vi "메인.vi"() -> ()   [LabVIEW 2021]
uses:
  <vilib>/Utility/miscctls.llb/LVPointTypeDef.ctl
  ctl/AI.ctl
  ctl/RS232.ctl
  ctl/DB.ctl
  ctl/SM.ctl
  ctl/CNN.ctl
  <vilib>/userDefined/High Color/IMAQdx.ctl
  <vilib>/Utility/sysdir.llb/System Directory Type.ctl
  <vilib>/DAQmx/read.llb/DAQmx Read (Analog 1D Wfm NChan NSamp).vi
  <vilib>/Analysis/baseanly.llb/Mean (DBL).vi
  <vilib>/Utility/file.llb/Write Delimited Spreadsheet (DBL).vi
  <vilib>/addons/database/Connection.llb/DB Tools Open Connec (String).vi
  <vilib>/Instr/_visa.llb/VISA Configure Serial Port (Instr).vi
  <vilib>/DAQmx/create/channels.llb/DAQmx Create Channel (AI-Voltage-Basic).vi
  <vilib>/DAQmx/configure/timing.llb/DAQmx Timing (Sample Clock).vi
  <vilib>/DAQmx/miscellaneous.llb/DAQmx Fill In Error Info.vi
  <vilib>/Analysis/NI_AALBase.lvlib
  <vilib>/vision/driver/NI_Vision_Acquisition_Software.lvlib
  <vilib>/addons/database/NI_Database_API.lvlib
panel:
  out "원소":i16 format="%.0f ℃"
  out "온도":i16(slide) scale=0.0..100.0
  out "Image 2":T1(plugin-control)
  in  "정지":bool
  in  "측정 시작":bool
  out "CNN Result":string[](array[string])
  out "Factory 상태":string
  in  "여러 열 리스트박스":i32(listbox)
  out "Image":T1(plugin-control)
  out "거리센서":waveform(dbl)(graph)
  out "기울기 그래프":waveform(dbl)[](graph)
  out "가속도 그래프":waveform(dbl)(graph)
  # "Smart Factory Management System"
  # "Factory State"
  # "Accelometer"
  # "Gradient"
  # "Distance"
  # "Object State"
  # "Temperature"
  # "Real Time Image"
  # "Captured Image"
  # "Result Table"
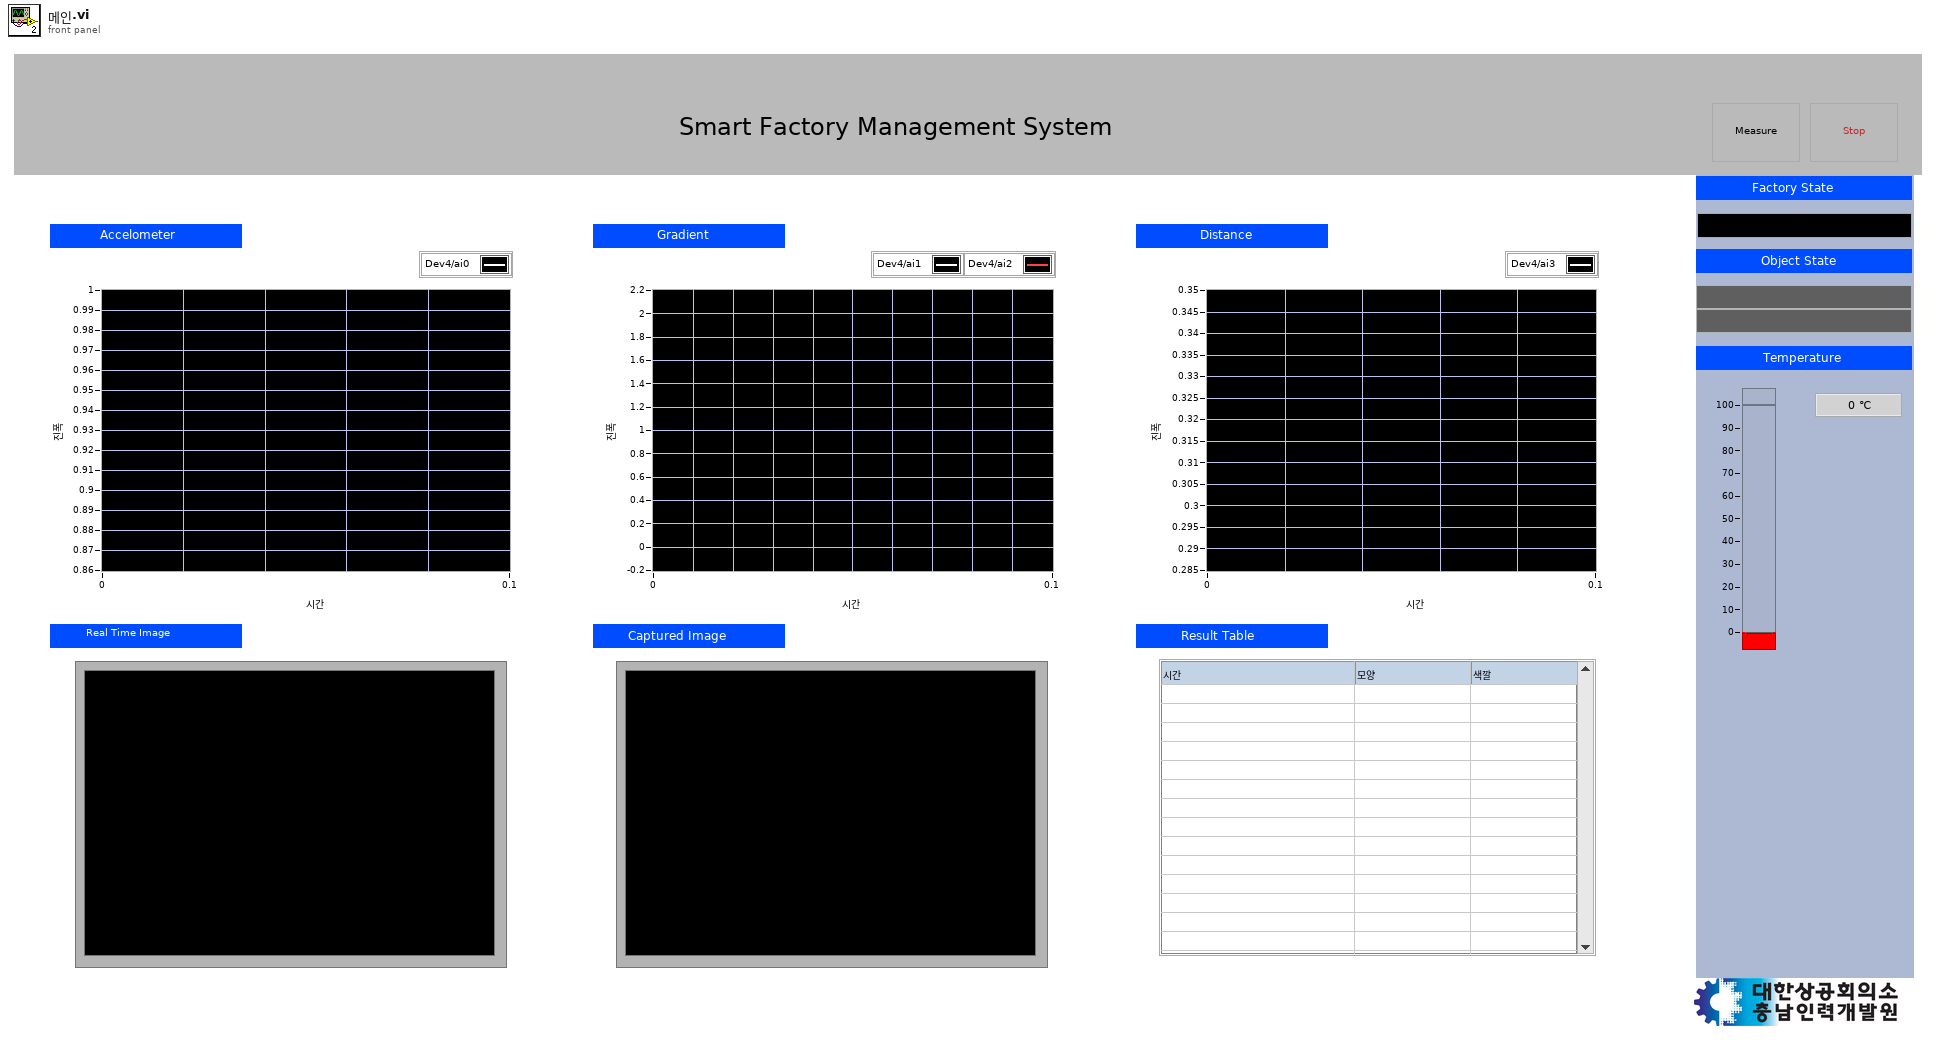
[diagram p1: front panel]
types:
  T1 = typedef "IMAQ Image.ctl" = refnum<image>
  T2 = typedef "LVPointTypeDef.ctl" = cluster{"Horizontal":i16, "Vertical":i16}
  T3 = cluster{"메인":refnum<queue>, "AI":refnum<queue>, "RS-232":refnum<queue>, "비전":refnum<queue>, "DB":refnum<queue>, "SM":refnum<queue>, "CNN":refnum<queue>}
  T4 = typedef "CNN.ctl" = cluster{"상태":enum16{"CNN 통신", "프로그램정지"}, "값":variant}
  T5 = typedef "SM.ctl" = cluster{"상태":enum16{"SM 통신", "프로그램정지"}, "값":variant}
  T6 = typedef "DB.ctl" = cluster{"상태":enum16{"초기화", "설정", "값 쓰기", "에러쓰기", "닫기", "프로그램정지"}, "값":variant}
  T7 = typedef "비전.ctl" = cluster{"상태":enum16{"초기화", "설정", "상시읽기", "트리거읽기", "닫기", "프로그램정지"}, "값":variant}
  T8 = typedef "RS232.ctl" = cluster{"상태":enum16{"초기화", "설정", "읽기", "닫기", "프로그램정지"}, "값":variant}
  T9 = typedef "AI.ctl" = cluster{"상태":enum16{"초기화", "설정", "읽기", "닫기", "프로그램정지"}, "값":variant}
  T10 = typedef "메인.ctl" = cluster{"상태":enum16{"초기화", "프로그램정지"}, "값":variant}
  T11 = enum16{"초기화", "설정", "값 쓰기", "에러쓰기", "닫기", "프로그램정지"}
  T12 = typedef "NI_Database_API.lvlib/Conn ObjectReference.ctl" = refnum<k1>
  T13 = cluster{"[0]":string, "[1]":string, "[2]":string}
  T14 = enum16{"Standard", "Buffered", "CRLF", "Immediate"}
  T15 = typedef "IMAQdx.ctl" = refnum<k21>
  T16 = enum16{"초기화", "설정", "상시읽기", "트리거읽기", "닫기", "프로그램정지"}
  T17 = typedef "System Directory Type.ctl" = i32
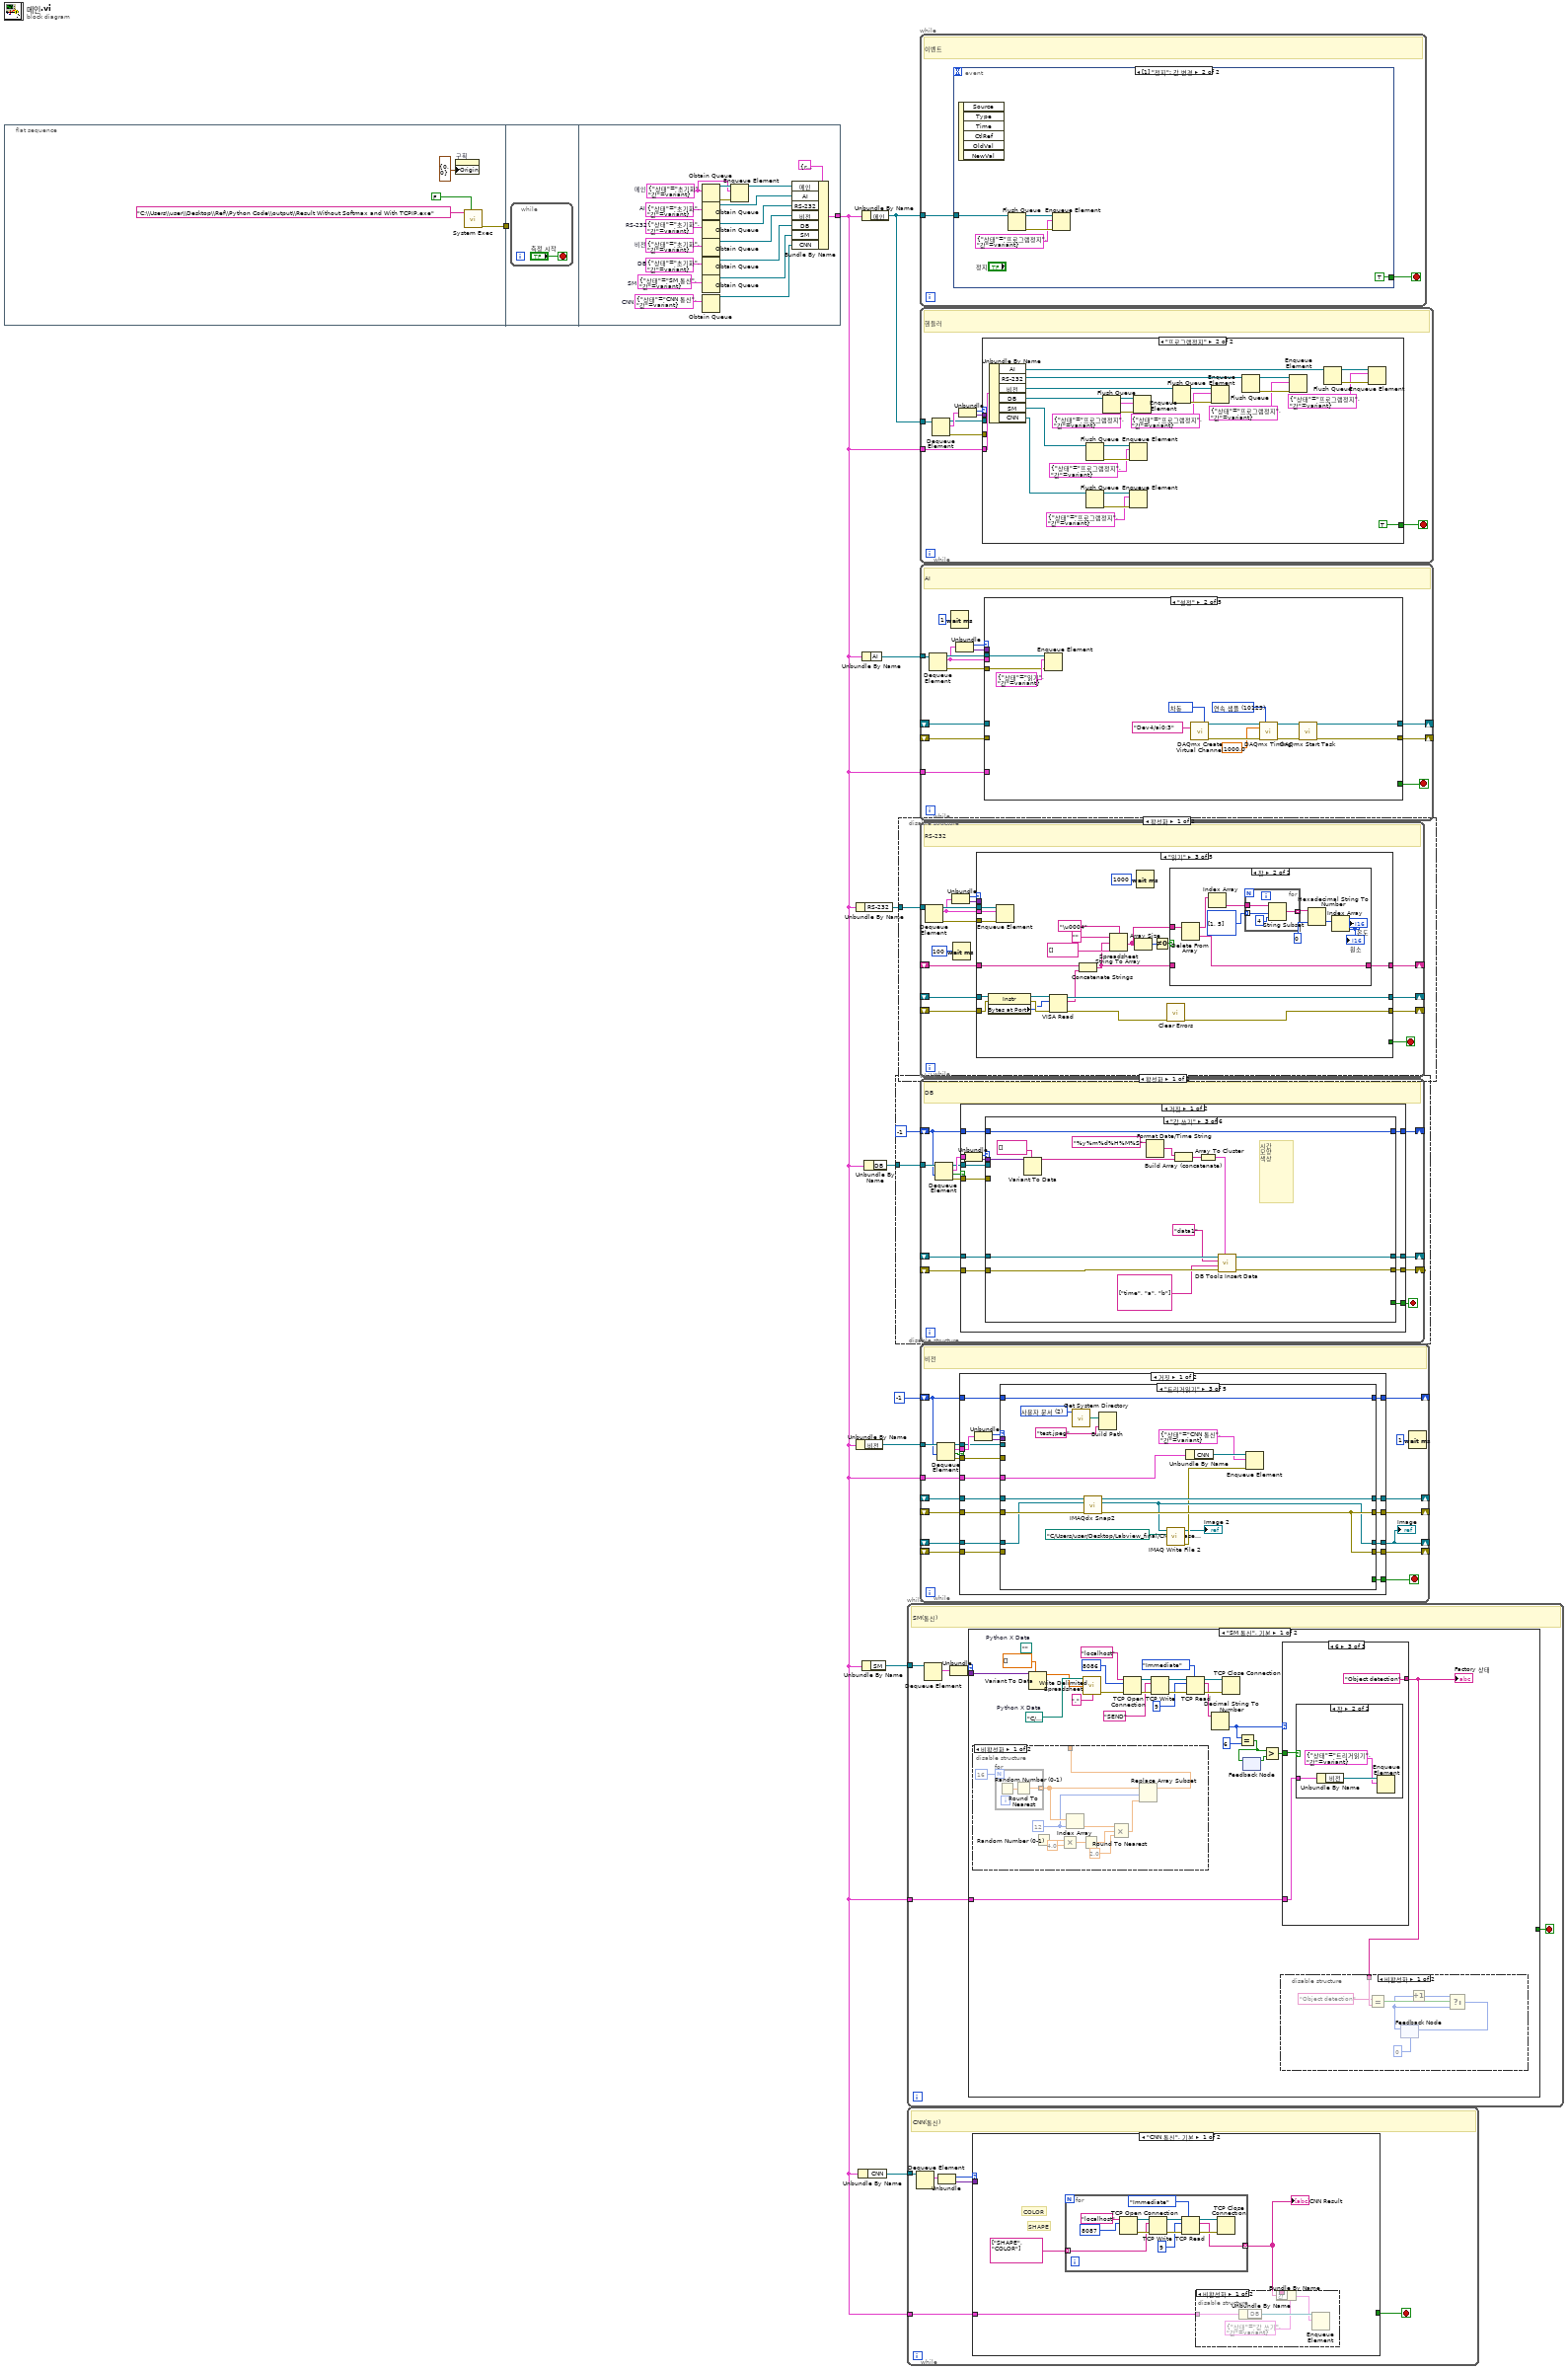
[diagram p0: block diagram]
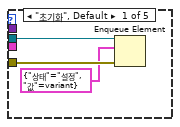
[diagram p2: hidden frame]
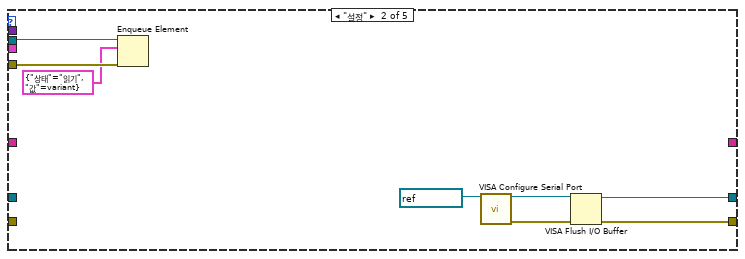
[diagram p3: hidden frame]
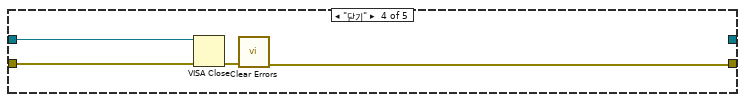
[diagram p5: hidden frame]
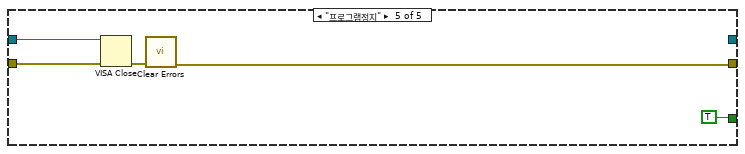
[diagram p6: hidden frame]
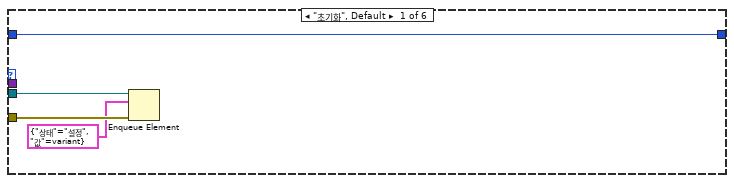
[diagram p8: hidden frame]
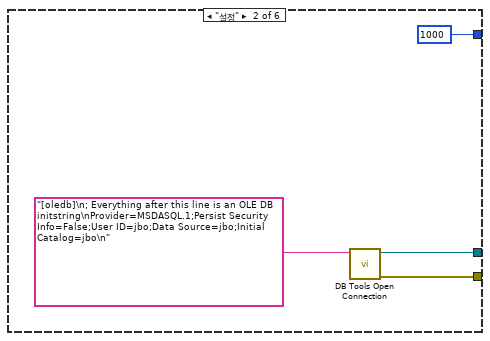
[diagram p9: hidden frame]
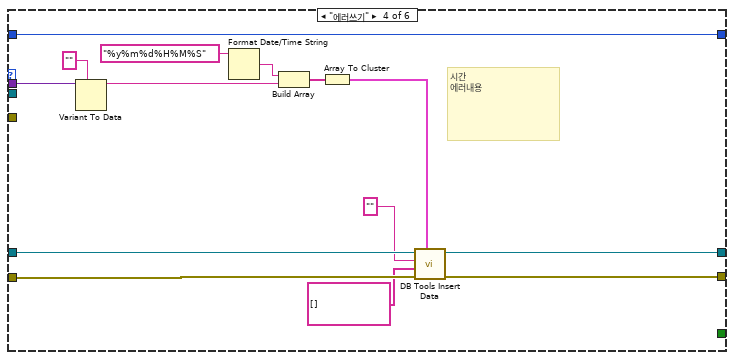
[diagram p10: hidden frame]
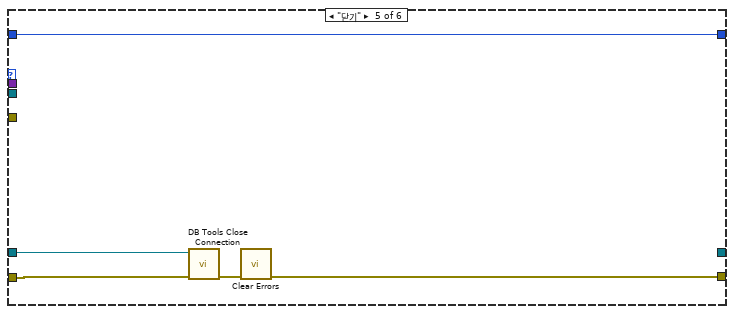
[diagram p11: hidden frame]
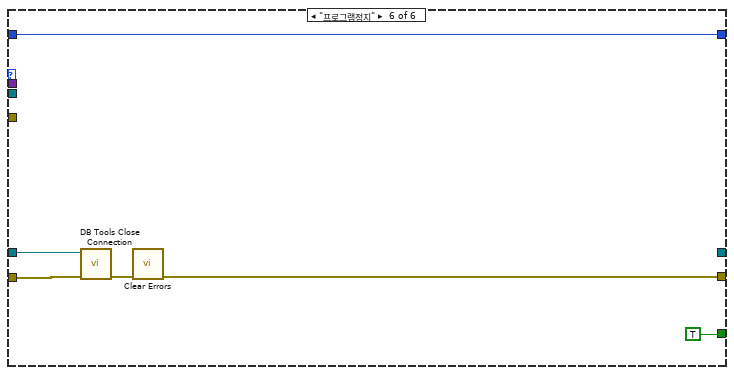
[diagram p12: hidden frame]
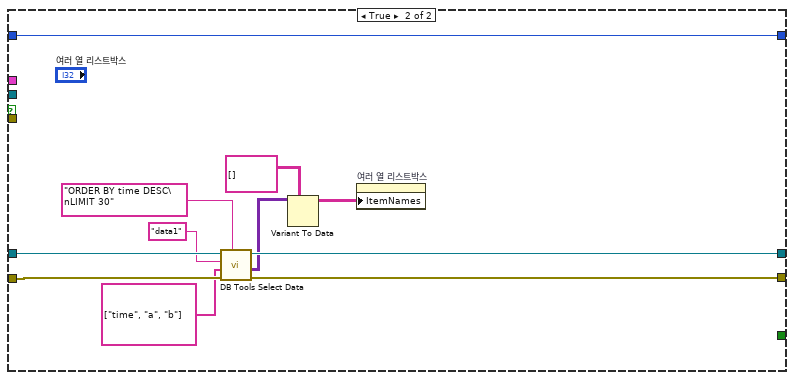
[diagram p13: hidden frame]
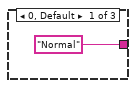
[diagram p17: hidden frame]
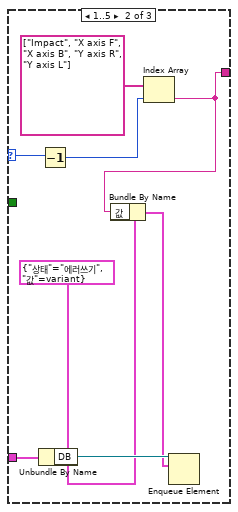
[diagram p18: hidden frame]
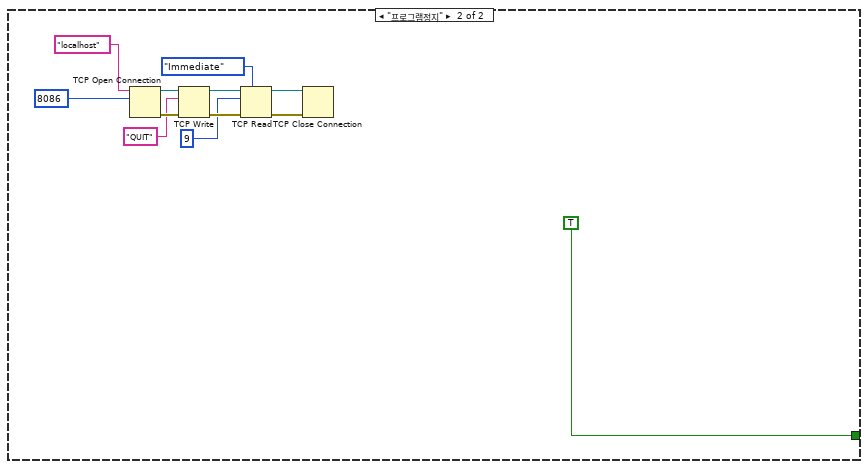
[diagram p20: hidden frame]
diagram:
  n1 = flat-sequence {
    tunnel: [w14] -> w1
    tunnel: w1 -> [_]
    tunnel: [w16] -> w2
    frame #0 {
      n2 = property on="구획" class="Pane"("Origin"=T2 {"Horizontal"=0, "Vertical"=0} ("원점")) -> ()  [unwired: 2 in, 2 out]
      n3 = call <vilib>:"System Exec.vi"("wait until completion? (T)"=FALSE, "command line"="C:\\Users\\user\\Desktop\\Ref\\Python Code\\output\\Result Without Softmax and With TCPIP.exe") -> ("error out"=w14:errorcluster)  [unwired: 6 in, 3 out]
    }
    frame #1 {
      n4 = while {
        stop <- "측정 시작" stop-if-true
      }
    }
    frame #2 {
      w19 = T4 {"상태"=enum."CNN 통신", "값"=variant}  # CNN
      w20 = T5 {"상태"=enum."SM 통신", "값"=variant}  # SM
      w30 = T6 {"상태"=enum."초기화", "값"=variant}  # DB
      w31 = T7 {"상태"=enum."초기화", "값"=variant}  # 비전
      w32 = T8 {"상태"=enum."초기화", "값"=variant}  # RS-232
      w33 = T9 {"상태"=enum."초기화", "값"=variant}  # AI
      w21 = T10 {"상태"=enum."초기화", "값"=variant}  # 메인
      n5 = Obtain Queue(element data type=w21) -> (queue out=w28:refnum<queue>, error out=w22:errorcluster)  [unwired: 4 in, 1 out]
      n6 = Obtain Queue(element data type=w33) -> (queue out=w27:refnum<queue>)  [unwired: 4 in, 2 out]
      n7 = Obtain Queue(element data type=w32) -> (queue out=w26:refnum<queue>)  [unwired: 4 in, 2 out]
      n8 = Obtain Queue(element data type=w31) -> (queue out=w25:refnum<queue>)  [unwired: 4 in, 2 out]
      n9 = Obtain Queue(element data type=w30) -> (queue out=w24:refnum<queue>)  [unwired: 4 in, 2 out]
      n10 = Obtain Queue(element data type=w20) -> (queue out=w18:refnum<queue>)  [unwired: 4 in, 2 out]
      n11 = Obtain Queue(element data type=w19) -> (queue out=w17:refnum<queue>)  [unwired: 4 in, 2 out]
      n12 = Enqueue Element(queue=w28, element=w21, error in (no error)=w22) -> (queue out=w23:refnum<queue>)  [unwired: 1 in, 2 out]
      n13 = Bundle By Name(cluster=T3 {"메인"=refnum, "AI"=refnum, "RS-232"=refnum, "비전"=refnum, "DB"=refnum, "SM"=refnum, "CNN"=refnum}, "메인"=w23, "AI"=w27, "RS-232"=w26, "비전"=w25, "DB"=w24, "SM"=w18, "CNN"=w17) -> (w16:T3)
    }
  }
  n14 = Unbundle By Name(w2) -> ("비전"=w6:refnum<queue>)
  n15 = Unbundle By Name(w2) -> ("RS-232"=w8:refnum<queue>)
  n16 = Unbundle By Name(w2) -> ("CNN"=w3:refnum<queue>)
  n17 = Unbundle By Name(w2) -> ("메인"=w10:refnum<queue>)
  n18 = Unbundle By Name(w2) -> ("AI"=w9:refnum<queue>)
  n19 = Unbundle By Name(w2) -> ("SM"=w4:refnum<queue>)
  n20 = Unbundle By Name(w2) -> ("DB"=w7:refnum<queue>)
  n21 = disable-structure shown="활성화" {
    disable-tunnel: w7 -> [w35 _]
    frame Enabled {
      n22 = while {
        tunnel: w35 -> [w46]
        shift-right: [w42] -> _
        shift-left: _ -> [w40]
        shift-right: [w41] -> _
        shift-left: _ -> [w39]
        shift-right: [w38] -> _
        shift-left: -1 -> [w37]
        stop <- w43 stop-if-true
        # "DB"
        n23 = Dequeue Element(queue=w46, timeout in ms (-1)=w37) -> (queue out=w45:refnum<queue>, element=w47:T6, timed out?=w36:bool, error out=w44:errorcluster)  [unwired: 1 in]
        n24 = case shown="거짓" w36 {
          tunnel: w47 -> [w59 _]
          tunnel: w45 -> [w56 _]
          tunnel: w44 -> [w55 _]
          tunnel: [w54 _] -> w43
          tunnel: [w53 w114] -> w42
          tunnel: [w52 w113] -> w41
          tunnel: w40 -> [w51 w116]
          tunnel: w39 -> [w50 w115]
          tunnel: [w49 w117] -> w38
          tunnel: w37 -> [w48 w117]
          frame False {
            n25 = Unbundle(w59) -> ("상태"=w58:T11, "값"=w57:variant)
            n26 = case shown="\"값 쓰기\"" w58 {
              tunnel: w57 -> [_ _ w77 w91 _ _]
              tunnel: w56 -> [w62 _ _ _ _ _]
              tunnel: w55 -> [w61 _ _ _ _ _]
              tunnel: [_ _ _ _ _ TRUE] -> w54
              tunnel: [_ w66 w79 w93 _ _] -> w53
              tunnel: [_ w65 w78 w92 w97 w102] -> w52
              tunnel: w51 -> [_ _ w81 w95 w100 w104]
              tunnel: w50 -> [_ _ w80 w94 w99 w103]
              tunnel: [w63 1000 w68 w82 w96 w101] -> w49
              tunnel: w48 -> [w63 _ w68 w82 w96 w101]
              frame "초기화", Default {
                n27 = Enqueue Element(queue=w62, element=T6 {"상태"=enum."설정", "값"=variant} ("원소"), error in (no error)=w61) -> ()  [unwired: 1 in, 3 out]
              }
              frame "설정" {
                n28 = call-poly <vilib>:"DB Tools Open Connection.vi"("connection information"="[oledb]\n; Everything after this line is an OLE DB initstring\nProvider=MSDASQL.1;Persist Security Info=False;User ID=jbo;Data Source=jbo;Initial Catalog=jbo\n") -> ("error out"=w65:errorcluster, "connection reference"=w66:T12)  [unwired: 7 in]
              }
              frame "값 쓰기" {
                # "시간\n모양\n색상"
                n29 = Variant To Data(type=string[] [], Variant=w77) -> (data=w71:string[])  [unwired: 1 in, 1 out]
                n30 = Format Date/Time String(time format string (%c)="%y%m%d%H%M%S" ("시간 포맷 문자열 (%c)")) -> (date/time string=w72:string)  [unwired: 2 in]
                n31 = Build Array (concatenate)(w72, w71) -> (w73:string[])
                n32 = Array To Cluster(array=w73) -> (cluster=w75:T13)
                n33 = call <vilib>:"DB Tools Insert Data.vi"("data"=w75, "error in (no error)"=w80, "columns"=string[] ["time", "a", "b"], "table"="data1", "connection reference"=w81) -> ("error out"=w78:errorcluster, "connection reference out"=w79:T12)  [unwired: 5 in]
              }
              frame "에러쓰기" {
                # "시간\n에러내용"
                n34 = Variant To Data(type="" ("숫자형"), Variant=w91) -> (data=w86:string)  [unwired: 1 in, 1 out]
                n35 = Format Date/Time String(time format string (%c)="%y%m%d%H%M%S" ("시간 포맷 문자열 (%c)")) -> (date/time string=w87:string)  [unwired: 2 in]
                n36 = Build Array(w87, w86) -> (w88:string[])
                n37 = Array To Cluster(array=w88) -> (cluster=w90:cluster{"[0]":string, "[1]":string})
                n38 = call <vilib>:"DB Tools Insert Data.vi"("data"=w90, "error in (no error)"=w94, "columns"=string[] [], "table"="", "connection reference"=w95) -> ("error out"=w92:errorcluster, "connection reference out"=w93:T12)  [unwired: 5 in]
              }
              frame "닫기" {
                n39 = call <vilib>:"DB Tools Close Connection.vi"("error in (no error)"=w99, "connection reference"=w100) -> ("error out"=w98:errorcluster)  [unwired: 5 in]
                n40 = call <vilib>:"Clear Errors.vi"("error in (no error)"=w98) -> ("error out"=w97:errorcluster)  [unwired: 5 in, 1 out]
              }
              frame "프로그램정지" {
                n41 = call <vilib>:"DB Tools Close Connection.vi"("error in (no error)"=w103, "connection reference"=w104) -> ("error out"=w105:errorcluster)  [unwired: 5 in]
                n42 = call <vilib>:"Clear Errors.vi"("error in (no error)"=w105) -> ("error out"=w102:errorcluster)  [unwired: 5 in, 1 out]
              }
            }
          }
          frame True {
            n43 = call <vilib>:"DB Tools Select Data.vi"("condition"="ORDER BY time DESC\nLIMIT 30", "error in (no error)"=w115, "columns"=string[] ["time", "a", "b"], "table"="data1", "connection reference"=w116) -> ("error out"=w113:errorcluster, "data"=w110:variant[][], "connection reference out"=w114:T12)  [unwired: 1 in]
            n44 = Variant To Data(type=string[][] [], Variant=w110) -> (data=w108:string[][])  [unwired: 1 in, 1 out]
            n45 = property on="여러 열 리스트박스" class="MCListbox (엄격한)"("ItemNames"=w108) -> ()  [unwired: 2 in, 2 out]
          }
        }
      }
    }
    frame Disabled {
    }
  }
  n46 = disable-structure shown="활성화" {
    disable-tunnel: w8 -> [w118 _]
    frame Enabled {
      n47 = while {
        tunnel: w118 -> [w132]
        shift-right: [w126] -> _
        shift-left: _ -> [w124]
        shift-right: [w125] -> _
        shift-left: _ -> [w123]
        shift-right: [w121] -> _
        shift-left: _ -> [w120]
        stop <- w127 stop-if-true
        # "RS-232"
        n48 = Dequeue Element(queue=w132) -> (queue out=w129:refnum<queue>, element=w122:T8, error out=w128:errorcluster)  [unwired: 2 in, 1 out]
        n49 = Unbundle(w122) -> ("상태"=w131:enum16{"초기화", "설정", "읽기", "닫기", "프로그램정지"}, "값"=w130:variant)
        n50 = Wait (ms)(milliseconds to wait=u32 100 ("대기 시간 (ms)")) -> ()  [unwired: 1 out]
        n51 = case shown="\"읽기\"" w131 {
          tunnel: w130 -> [_ _ _ _ _]
          tunnel: w129 -> [w135 w138 w158 _ _]
          tunnel: w128 -> [w134 w137 w157 _ _]
          tunnel: [_ _ _ _ TRUE] -> w127
          tunnel: [_ w141 w165 _ _] -> w126
          tunnel: [_ w140 w144 w180 w184] -> w125
          tunnel: w124 -> [_ _ w162 w183 w186]
          tunnel: w123 -> [_ _ w163 w182 w185]
          tunnel: w122 -> [_ _ w156 _ _]
          tunnel: [_ _ w147 _ _] -> w121
          tunnel: w120 -> [_ _ w146 _ _]
          frame "초기화", Default {
            n52 = Enqueue Element(queue=w135, element=T8 {"상태"=enum."설정", "값"=variant} ("원소"), error in (no error)=w134) -> ()  [unwired: 1 in, 3 out]
          }
          frame "설정" {
            n53 = Enqueue Element(queue=w138, element=T8 {"상태"=enum."읽기", "값"=variant} ("원소"), error in (no error)=w137) -> ()  [unwired: 1 in, 3 out]
            n54 = call-poly "VISA Configure Serial Port"("VISA resource name"=refnum<visa-resource-name> "COM6") -> ("VISA resource name out"=w143:refnum<visa-resource-name>, "error out"=w142:errorcluster)  [unwired: 13 in]
            n55 = VISA Flush I/O Buffer(VISA resource name=w143, error in (no error)=w142) -> (VISA resource name out=w141:refnum<visa-resource-name>, error out=w140:errorcluster)  [unwired: 1 in]
          }
          frame "읽기" {
            n56 = property class="Instr"(reference=w162, error in=w163) -> (reference out=w161:refnum<visa-resource-name>, error out=w160:errorcluster, "Bytes at Port"=w159:u32)
            n57 = Enqueue Element(queue=w158, element=w156, error in (no error)=w157) -> ()  [unwired: 1 in, 3 out]
            n58 = VISA Read(VISA resource name=w161, byte count=w159, error in (no error)=w160) -> (VISA resource name out=w165:refnum<visa-resource-name>, read buffer=w154:string, error out=w164:errorcluster)  [unwired: 1 out]
            n59 = Concatenate Strings(w146, w154) -> (w145:string)
            n60 = Spreadsheet String To Array(delimiter (Tab)="\u0004" ("구분 문자 (탭)"), format string="" ("포맷 문자열"), spreadsheet string=w145, array type (2D Dbl)=string[] [] ("포맷 문자열")) -> (array=w148:string[])
            n61 = Array Size(array=w148) -> (size(s)=w150:i32)
            n62 = Wait (ms)(milliseconds to wait=u32 1000 ("대기 시간 (ms)")) -> ()  [unwired: 1 out]
            n63 = Not Equal To 0?(x=w150) -> (x != 0?=w149:bool)
            n64 = call <vilib>:"Clear Errors.vi"("error in (no error)"=w164) -> ("error out"=w144:errorcluster)  [unwired: 5 in, 1 out]
            n65 = case shown="참" w149 {
              tunnel: w148 -> [_ w175]
              tunnel: [w166 w174] -> w147
              tunnel: w145 -> [w166 _]
              frame False {
              }
              frame True {
                n66 = Delete From Array(array=w175) -> (deleted portion=w174:string, array with subset deleted=w173:string[])  [unwired: 2 in]
                n67 = Index Array(array=w173) -> (element=w172:string)  [unwired: 1 in]
                n68 = for {
                  tunnel: w172 -> [w179]
                  tunnel: i32[] [1, 5] ("오프셋(0)") -> [w177] mode=indexing
                  tunnel: [w176] -> w170 mode=indexing
                  n69 = String Subset(string=w179, offset (0)=w177, length (rest)=4 ("길이(나머지)")) -> (substring=w176:string)
                }
                n70 = Hexadecimal String To Number(string=w170, default (0uL)=i16 0) -> (number=w168:i16[])  [unwired: 1 in, 1 out]
                n71 = Index Array(array=w168) -> (element=→"온도" →"원소":i16)  [unwired: 1 in]
              }
            }
          }
          frame "닫기" {
            n72 = VISA Close(VISA resource name=w183, error in (no error)=w182) -> (error out=w181:errorcluster)
            n73 = call <vilib>:"Clear Errors.vi"("error in (no error)"=w181) -> ("error out"=w180:errorcluster)  [unwired: 5 in, 1 out]
          }
          frame "프로그램정지" {
            n74 = VISA Close(VISA resource name=w186, error in (no error)=w185) -> (error out=w187:errorcluster)
            n75 = call <vilib>:"Clear Errors.vi"("error in (no error)"=w187) -> ("error out"=w184:errorcluster)  [unwired: 5 in, 1 out]
          }
        }
      }
    }
    frame Disabled {
    }
  }
  n76 = while {
    tunnel: w4 -> [w194]
    tunnel: w2 -> [w189]
    stop <- w190 stop-if-true
    # "SM(통신)"
    n77 = Dequeue Element(queue=w194) -> (element=w193:T5)  [unwired: 2 in, 3 out]
    n78 = Unbundle(w193) -> ("상태"=w192:enum16{"SM 통신", "프로그램정지"}, "값"=w191:variant)
    n79 = case shown="\"SM 통신\", 기본" w192 {
      tunnel: w191 -> [w219 _]
      tunnel: [_ TRUE] -> w190
      tunnel: w189 -> [w217 _]
      frame "SM 통신", Default {
        w199 = path "C:/Users/user/Desktop/Labview_final/Project/Data/Softmax/Test/x data4.csv"  # Python X Data
        (unwired) path ""  # Python X Data
        n80 = disable-structure shown="비활성화" {
          disable-tunnel: [w220 _] -> _
          frame Disabled {
            w223 = 12 ("인덱스")
            n81 = for {
              N: 16 -> [_]
              tunnel: [w231] -> w225 mode=indexing
              n82 = Random Number (0-1)() -> (number: 0 to 1=w232:dbl)
              n83 = Round To Nearest(number=w232) -> (nearest integer value=w231:dbl)
            }
            n84 = Random Number (0-1)() -> (number: 0 to 1=w230:dbl)
            n85 = Multiply(x=w230, y=4.0) -> (x*y=w228:dbl)
            n86 = Index Array(array=w225, index=w223) -> (element=w226:dbl)
            n87 = Round To Nearest(number=w228) -> (nearest integer value=w227:dbl)
            n88 = Compound Arithmetic op=MULTIPLY(w226, w227, 2.0 ("값")) -> (w224:dbl)
            n89 = Replace Array Subset(array=w225, new element=w224, index=w223) -> (w220:dbl[])
          }
          frame Enabled {
          }
        }
        n90 = Variant To Data(type=dbl[] [], Variant=w219) -> (data=w195:dbl[])  [unwired: 1 in, 1 out]
        n91 = call-poly <vilib>:"Write Delimited Spreadsheet.vi"("file path (dialog if empty)"=w199, "1D data"=w195, "delimiter (\\t)"="," ("delimiter (\\t)")) -> ("error out"=w212:errorcluster)  [unwired: 11 in, 1 out]
        n92 = TCP Open Connection(address="localhost" ("주소"), remote port or service name=u16 8086 ("원격 포트 또는 서비스 이름"), error in (no error)=w212) -> (connection ID=w208:refnum<k5>, error out=w211:errorcluster)  [unwired: 2 in]
        n93 = TCP Write(connection ID=w208, data in="SEND" ("데이터 입력"), error in (no error)=w211) -> (connection ID out=w207:refnum<k5>, error out=w210:errorcluster)  [unwired: 1 in, 1 out]
        n94 = TCP Read(connection ID=w207, bytes to read=9 ("읽을 바이트"), error in (no error)=w210, 7:T14."Immediate" ("모드(standard)")) -> (connection ID out=w206:refnum<k5>, data out=w200:string, error out=w209:errorcluster)  [unwired: 1 in]
        n95 = Decimal String To Number(string=w200) -> (number=w196:i32)  [unwired: 2 in, 1 out]
        n96 = TCP Close Connection(connection ID=w206, error in (no error)=w209) -> ()  [unwired: 1 in, 2 out]
        n97 = Equal?(x=w196, y=6) -> (x = y?=w215:bool)
        n98 = feedback-in #1(w215) -> ()
        n99 = feedback #1() -> (w214:bool)  [unwired: 1 in]
        n100 = Greater?(x=w215, y=w214) -> (0:w213:bool)
        n101 = case shown="6" w196 {
          selector: w196 -> [_ w247 _]
          tunnel: ["Normal" w241 "Object detection"] -> w197
          tunnel: w217 -> [_ w245 w249]
          tunnel: w213 -> [_ _ w250]
          frame 0, Default {
          }
          frame 1..5 {
            n102 = Unbundle By Name(w245) -> ("DB"=w244:refnum<queue>)
            n103 = Decrement(x=w247) -> (x-1=w246:i32)
            n104 = Index Array(array=string[] ["Impact", "X axis F", "X axis B", "Y axis R", "Y axis L"], index=w246) -> (element=w241:string)
            n105 = Bundle By Name(cluster=T6 {"상태"=enum."에러쓰기", "값"=variant} ("원소"), "값"=w241) -> (w242:T6)
            n106 = Enqueue Element(queue=w244, element=w242) -> ()  [unwired: 2 in, 3 out]
          }
          frame 6 {
            n107 = case shown="참" w250 {
              tunnel: w249 -> [_ w254]
              frame False {
              }
              frame True {
                n108 = Unbundle By Name(w254) -> ("비전"=w253:refnum<queue>)
                n109 = Enqueue Element(queue=w253, element=T7 {"상태"=enum."트리거읽기", "값"=variant} ("원소")) -> ()  [unwired: 2 in, 3 out]
              }
            }
          }
        }
        "Factory 상태" <- w197
        n110 = disable-structure shown="비활성화" {
          disable-tunnel: w197 -> [w239 _]
          frame Disabled {
            n111 = Equal?(x="Object detection", y=w239) -> (x = y?=w237:bool)
            n112 = feedback #2(0) -> (w235:i32)
            n113 = Increment(x=w235) -> (x+1=w234:i32)
            n114 = Select(t=w234, s=w237, f=w235) -> (s? t:f=w233:i32)
            n115 = feedback-in #2(w233) -> ()
          }
          frame Enabled {
          }
        }
      }
      frame "프로그램정지" {
        n116 = TCP Open Connection(address="localhost" ("주소"), remote port or service name=u16 8086 ("원격 포트 또는 서비스 이름")) -> (connection ID=w262:refnum<k5>, error out=w265:errorcluster)  [unwired: 3 in]
        n117 = TCP Write(connection ID=w262, data in="QUIT" ("데이터 입력"), error in (no error)=w265) -> (connection ID out=w261:refnum<k5>, error out=w264:errorcluster)  [unwired: 1 in, 1 out]
        n118 = TCP Read(connection ID=w261, bytes to read=9 ("읽을 바이트"), error in (no error)=w264, 7:T14."Immediate" ("모드(standard)")) -> (connection ID out=w260:refnum<k5>, error out=w263:errorcluster)  [unwired: 1 in, 1 out]
        n119 = TCP Close Connection(connection ID=w260, error in (no error)=w263) -> ()  [unwired: 1 in, 2 out]
      }
    }
  }
  n120 = while {
    tunnel: w3 -> [w272]
    tunnel: w2 -> [w268]
    stop <- w267 stop-if-true
    # "CNN(통신)"
    n121 = Dequeue Element(queue=w272) -> (element=w271:T4)  [unwired: 2 in, 3 out]
    n122 = Unbundle(w271) -> ("상태"=w270:enum16{"CNN 통신", "프로그램정지"}, "값"=w269:variant)
    n123 = case shown="\"CNN 통신\", 기본" w270 {
      tunnel: w269 -> [_ _]
      tunnel: w268 -> [w275 _]
      tunnel: [_ TRUE] -> w267
      frame "CNN 통신", Default {
        # "SHAPE"
        # "COLOR"
        n124 = for {
          tunnel: string[] ["SHAPE", "COLOR"] -> [w279] mode=indexing
          tunnel: [w277] -> w274 mode=indexing
          n125 = TCP Open Connection(address="localhost" ("주소"), remote port or service name=u16 8087 ("원격 포트 또는 서비스 이름")) -> (connection ID=w284:refnum<k5>, error out=w287:errorcluster)  [unwired: 3 in]
          n126 = TCP Write(connection ID=w284, data in=w279, error in (no error)=w287) -> (connection ID out=w283:refnum<k5>, error out=w286:errorcluster)  [unwired: 1 in, 1 out]
          n127 = TCP Read(connection ID=w283, bytes to read=9 ("읽을 바이트"), error in (no error)=w286, 7:T14."Immediate" ("모드(standard)")) -> (connection ID out=w282:refnum<k5>, data out=w277:string, error out=w285:errorcluster)  [unwired: 1 in]
          n128 = TCP Close Connection(connection ID=w282, error in (no error)=w285) -> ()  [unwired: 1 in, 2 out]
        }
        "CNN Result" <- w274
        n129 = disable-structure shown="비활성화" {
          disable-tunnel: w275 -> [w292 _]
          disable-tunnel: w274 -> [w288 _]
          frame Disabled {
            n130 = Unbundle By Name(w292) -> ("DB"=w291:refnum<queue>)
            n131 = Bundle By Name(cluster=T6 {"상태"=enum."값 쓰기", "값"=variant} ("원소"), "값"=w288) -> (w289:T6)
            n132 = Enqueue Element(queue=w291, element=w289) -> ()  [unwired: 2 in, 3 out]
          }
          frame Enabled {
          }
        }
      }
      frame "프로그램정지" {
        n133 = TCP Open Connection(address="localhost" ("주소"), remote port or service name=u16 8087 ("원격 포트 또는 서비스 이름")) -> (connection ID=w300:refnum<k5>, error out=w303:errorcluster)  [unwired: 3 in]
        n134 = TCP Write(connection ID=w300, data in="QUIT" ("데이터 입력"), error in (no error)=w303) -> (connection ID out=w299:refnum<k5>, error out=w302:errorcluster)  [unwired: 1 in, 1 out]
        n135 = TCP Read(connection ID=w299, bytes to read=9 ("읽을 바이트"), error in (no error)=w302, 7:T14."Immediate" ("모드(standard)")) -> (connection ID out=w298:refnum<k5>, error out=w301:errorcluster)  [unwired: 1 in, 1 out]
        n136 = TCP Close Connection(connection ID=w298, error in (no error)=w301) -> ()  [unwired: 1 in, 2 out]
      }
    }
  }
  n137 = while {
    tunnel: w10 -> [w305]
    stop <- w306 stop-if-true
    # "이벤트"
    n138 = event shown="[1] \"정지\": 값 변경" {
      selector: _ -> [_ _]
      dyn-events: _ -> [_ _]
      timeout: _ -> [_ _]
      tunnel: [w311 TRUE ("버림?")] -> w306
      tunnel: w305 -> [w308 w314]
      event Panel Close? {
        w311 = TRUE ("버림?")
        n139 = event-data() -> ()  [unwired: 1 in, 4 out]
        n140 = Flush Queue(queue=w308) -> (queue out=w309:refnum<queue>, error out=w310:errorcluster)  [unwired: 1 in, 1 out]
        n141 = Enqueue Element(queue=w309, element=T10 {"상태"=enum."프로그램정지", "값"=variant} ("원소"), error in (no error)=w310) -> ()  [unwired: 1 in, 3 out]
        n142 = event-data("Discard?"=w311) -> ()  [unwired: 1 in, 1 out]
      }
      event "정지": Value Change {
        n143 = event-data() -> ()  [unwired: 1 in, 6 out]
        n144 = Flush Queue(queue=w314) -> (queue out=w315:refnum<queue>, error out=w316:errorcluster)  [unwired: 1 in, 1 out]
        n145 = Enqueue Element(queue=w315, element=T10 {"상태"=enum."프로그램정지", "값"=variant} ("원소"), error in (no error)=w316) -> ()  [unwired: 1 in, 3 out]
      }
    }
  }
  n146 = while {
    tunnel: w2 -> [w324]
    tunnel: w10 -> [w323]
    stop <- w317 stop-if-true
    # "헨들러"
    n147 = Dequeue Element(queue=w323) -> (queue out=w321:refnum<queue>, element=w322:T10, error out=w318:errorcluster)  [unwired: 2 in, 1 out]
    n148 = Unbundle(w322) -> ("상태"=w320:enum16{"초기화", "프로그램정지"}, "값"=w319:variant)
    n149 = case shown="\"프로그램정지\"" w320 {
      tunnel: w324 -> [w329 w343]
      tunnel: w321 -> [_ _]
      tunnel: w319 -> [_ _]
      tunnel: w318 -> [_ _]
      tunnel: [_ TRUE] -> w317
      frame "초기화", Default {
        n150 = Unbundle By Name(w329) -> ("AI"=w328:refnum<queue>, "RS-232"=w327:refnum<queue>, "비전"=w326:refnum<queue>, "DB"=w325:refnum<queue>)
        n151 = Enqueue Element(queue=w325, element=T6 {"상태"=enum."초기화", "값"=variant} ("원소")) -> ()  [unwired: 2 in, 3 out]
        n152 = Enqueue Element(queue=w326, element=T7 {"상태"=enum."초기화", "값"=variant} ("원소")) -> ()  [unwired: 2 in, 3 out]
        n153 = Enqueue Element(queue=w327, element=T8 {"상태"=enum."초기화", "값"=variant} ("원소")) -> ()  [unwired: 2 in, 3 out]
        n154 = Enqueue Element(queue=w328, element=T9 {"상태"=enum."초기화", "값"=variant} ("원소")) -> ()  [unwired: 2 in, 3 out]
      }
      frame "프로그램정지" {
        n155 = Unbundle By Name(w343) -> ("AI"=w352:refnum<queue>, "RS-232"=w353:refnum<queue>, "비전"=w359:refnum<queue>, "DB"=w358:refnum<queue>, "SM"=w339:refnum<queue>, "CNN"=w335:refnum<queue>)
        n156 = Flush Queue(queue=w339) -> (queue out=w341:refnum<queue>, error out=w340:errorcluster)  [unwired: 1 in, 1 out]
        n157 = Flush Queue(queue=w335) -> (queue out=w337:refnum<queue>, error out=w336:errorcluster)  [unwired: 1 in, 1 out]
        n158 = Flush Queue(queue=w358) -> (queue out=w355:refnum<queue>, error out=w354:errorcluster)  [unwired: 1 in, 1 out]
        n159 = Enqueue Element(queue=w341, element=T5 {"상태"=enum."프로그램정지", "값"=variant} ("원소"), error in (no error)=w340) -> ()  [unwired: 1 in, 3 out]
        n160 = Enqueue Element(queue=w337, element=T4 {"상태"=enum."프로그램정지", "값"=variant} ("원소"), error in (no error)=w336) -> ()  [unwired: 1 in, 3 out]
        n161 = Enqueue Element(queue=w355, element=T6 {"상태"=enum."프로그램정지", "값"=variant} ("원소"), error in (no error)=w354) -> ()  [unwired: 1 in, 3 out]
        n162 = Flush Queue(queue=w359) -> (queue out=w356:refnum<queue>, error out=w357:errorcluster)  [unwired: 1 in, 1 out]
        n163 = Enqueue Element(queue=w356, element=T7 {"상태"=enum."프로그램정지", "값"=variant} ("원소"), error in (no error)=w357) -> ()  [unwired: 1 in, 3 out]
        n164 = Flush Queue(queue=w353) -> (queue out=w350:refnum<queue>, error out=w351:errorcluster)  [unwired: 1 in, 1 out]
        n165 = Enqueue Element(queue=w350, element=T8 {"상태"=enum."프로그램정지", "값"=variant} ("원소"), error in (no error)=w351) -> ()  [unwired: 1 in, 3 out]
        n166 = Flush Queue(queue=w352) -> (queue out=w349:refnum<queue>, error out=w348:errorcluster)  [unwired: 1 in, 1 out]
        n167 = Enqueue Element(queue=w349, element=T9 {"상태"=enum."프로그램정지", "값"=variant} ("원소"), error in (no error)=w348) -> ()  [unwired: 1 in, 3 out]
      }
    }
  }
  n168 = while {
    tunnel: w9 -> [w372]
    shift-right: [w366] -> _
    shift-left: _ -> [w364]
    shift-right: [w365] -> _
    shift-left: _ -> [w363]
    tunnel: w2 -> [w360]
    stop <- w368 stop-if-true
    # "AI"
    n169 = Dequeue Element(queue=w372) -> (queue out=w370:refnum<queue>, element=w362:T9, error out=w369:errorcluster)  [unwired: 2 in, 1 out]
    n170 = Wait (ms) ("기다림(ms)")(milliseconds to wait=u32 1 ("대기 시간 (ms)")) -> ()  [unwired: 1 out]
    n171 = Unbundle(w362) -> ("상태"=w371:enum16{"초기화", "설정", "읽기", "닫기", "프로그램정지"}, "값"=w367:variant)
    n172 = case shown="\"설정\"" w371 {
      tunnel: w370 -> [w375 w378 w397 _ _]
      tunnel: w369 -> [w374 w377 w396 _ _]
      tunnel: [_ _ _ _ TRUE] -> w368
      tunnel: w367 -> [_ _ _ _ _]
      tunnel: [_ w385 w410 _ _] -> w366
      tunnel: [errorcluster {"status"=FALSE, "code"=0, "source"=""} ("error out") w384 w409 w416 w420] -> w365
      tunnel: w364 -> [_ _ w412 w419 w422]
      tunnel: w363 -> [_ _ w411 w418 w421]
      tunnel: w362 -> [_ _ w395 _ _]
      tunnel: w360 -> [_ _ w394 _ _]
      frame "초기화", Default {
        n173 = Enqueue Element(queue=w375, element=T9 {"상태"=enum."설정", "값"=variant} ("원소"), error in (no error)=w374) -> ()  [unwired: 1 in, 3 out]
      }
      frame "설정" {
        w381 = 10123 items=["유한 샘플"=10178, "연속 샘플"=10123, "하드웨어 타이밍에 의한 단일 포인트"=12522] ("sample mode")
        w382 = 10106 items=["기본"=-1, "RSE"=10083, "NRSE"=10078, "차동"=10106, "유사 차동"=12529] ("input terminal configuration")
        n174 = Enqueue Element(queue=w378, element=T9 {"상태"=enum."읽기", "값"=variant} ("원소"), error in (no error)=w377) -> ()  [unwired: 1 in, 3 out]
        n175 = call-poly <vilib>:"DAQmx Create Virtual Channel.vi"("input terminal configuration"=w382, "physical channels"=tag "Dev4/ai0:3") -> ("task out"=w389:refnum<k21>, "error out"=w388:errorcluster)  [unwired: 12 in]
        n176 = call-poly <vilib>:"DAQmx Timing.vi"("task/channels in"=w389, "sample mode"=w381, "rate"=1000.0, "error in"=w388) -> ("task out"=w387:refnum<k21>, "error out"=w386:errorcluster)  [unwired: 10 in]
        n177 = call <vilib>:"DAQmx Start Task.vi"("task/channels in"=w387, "error in"=w386) -> ("task out"=w385:refnum<k21>, "error out"=w384:errorcluster)  [unwired: 12 in]
      }
      frame "읽기" {
        n178 = Enqueue Element(queue=w397, element=w395, error in (no error)=w396) -> ()  [unwired: 1 in, 3 out]
        n179 = call-poly <vilib>:"DAQmx Read.vi"("task/channels in"=w412, "number of samples per channel"=100, "error in"=w411) -> ("task out"=w410:refnum<k21>, "data"=w407:waveform(dbl)[], "error out"=w409:errorcluster)  [unwired: 10 in]
        n180 = Subtract(x=w407, y=dbl[] [2.5, 2.5, 2.5, 0.0]) -> (x-y=w405:waveform(dbl)[])
        n181 = Multiply(x=w405, y=dbl[] [4.0, 30.0, 30.0, 1.0]) -> (x*y=w398:waveform(dbl)[])
        n182 = Index Array(array=w398) -> (element #1=→"가속도 그래프":waveform(dbl), element #2=w403:waveform(dbl), element #3=w402:waveform(dbl), element #4=→"거리센서":waveform(dbl))  [unwired: 4 in]
        n183 = for {
          tunnel: w398 -> [w415] mode=indexing
          tunnel: [w413] -> w391 mode=indexing
          n184 = Unbundle By Name(w415) -> ("Y"=w414:dbl[])
          n185 = call-poly <vilib>:"Mean.vi"("X"=w414) -> ("mean"=w413:dbl)  [unwired: 1 out]
        }
        n186 = Unbundle By Name(w394) -> ("SM"=w393:refnum<queue>)
        n187 = Build Array(w403, w402) -> (→"기울기 그래프":waveform(dbl)[])
        n188 = Bundle By Name(cluster=T5 {"상태"=enum."SM 통신", "값"=variant} ("원소"), "값"=w391) -> (w390:T5)
        n189 = Enqueue Element(queue=w393, element=w390) -> ()  [unwired: 2 in, 3 out]
      }
      frame "닫기" {
        n190 = call <vilib>:"DAQmx Clear Task.vi"("task in"=w419, "error in"=w418) -> ("error out"=w417:errorcluster)  [unwired: 13 in]
        n191 = call <vilib>:"Clear Errors.vi"("error in (no error)"=w417) -> ("error out"=w416:errorcluster)  [unwired: 5 in, 1 out]
      }
      frame "프로그램정지" {
        n192 = call <vilib>:"DAQmx Clear Task.vi"("task in"=w422, "error in"=w421) -> ("error out"=w423:errorcluster)  [unwired: 13 in]
        n193 = call <vilib>:"Clear Errors.vi"("error in (no error)"=w423) -> ("error out"=w420:errorcluster)  [unwired: 5 in, 1 out]
      }
    }
  }
  n194 = while {
    tunnel: w6 -> [w441]
    shift-right: [w437] -> _
    shift-left: _ -> [w434]
    shift-right: [w436] -> _
    shift-left: _ -> [w433]
    shift-right: [w427] -> _
    shift-left: _ -> [w432]
    shift-right: [w435] -> _
    shift-left: _ -> [w431]
    shift-right: [w430] -> _
    shift-left: -1 -> [w429]
    tunnel: w2 -> [w425]
    stop <- w438 stop-if-true
    # "비전"
    n195 = Dequeue Element(queue=w441, timeout in ms (-1)=w429) -> (queue out=w440:refnum<queue>, element=w442:T7, timed out?=w428:bool, error out=w439:errorcluster)  [unwired: 1 in]
    n196 = case shown="거짓" w428 {
      tunnel: w442 -> [w459 _]
      tunnel: w440 -> [w456 _]
      tunnel: w439 -> [w455 _]
      tunnel: [w454 _] -> w438
      tunnel: [w453 w510] -> w437
      tunnel: [w452 w506] -> w436
      tunnel: [w451 w507] -> w427
      tunnel: [w450 w506] -> w435
      tunnel: w434 -> [w449 w511]
      tunnel: w433 -> [w448 w509]
      tunnel: w432 -> [w447 w508]
      tunnel: w431 -> [w446 _]
      tunnel: [w445 w512] -> w430
      tunnel: w429 -> [w444 w512]
      tunnel: w425 -> [w443 _]
      frame False {
        n197 = Unbundle(w459) -> ("상태"=w458:T16, "값"=w457:variant)
        n198 = case shown="\"트리거읽기\"" w458 {
          tunnel: w457 -> [_ _ _ _ _]
          tunnel: w456 -> [w463 _ _ _ _]
          tunnel: w455 -> [w462 _ _ _ _]
          tunnel: [_ _ _ _ TRUE] -> w454
          tunnel: [_ w470 w482 _ _] -> w453
          tunnel: [_ w469 w481 w489 w497] -> w452
          tunnel: [_ w468 w480 _ _] -> w451
          tunnel: [_ w467 w481 w487 w496] -> w450
          tunnel: w449 -> [_ _ w485 w494 w501]
          tunnel: w448 -> [_ _ w484 w493 w500]
          tunnel: w447 -> [_ _ w483 w492 w499]
          tunnel: w446 -> [_ _ _ w491 w498]
          tunnel: [w460 100 w486 w495 w504] -> w445
          tunnel: w444 -> [w460 _ w486 w495 w504]
          tunnel: w443 -> [_ _ w476 _ _]
          frame "초기화", Default {
            n199 = Enqueue Element(queue=w463, element=T7 {"상태"=enum."설정", "값"=variant} ("원소"), error in (no error)=w462) -> ()  [unwired: 1 in, 3 out]
          }
          frame "설정" {
            n200 = call <vilib>:"IMAQdx Open Camera.vi"("Session In"=T15 "cam2") -> ("error out"=w469:errorcluster, "Session Out"=w470:T15)  [unwired: 9 in]
            n201 = call "IMAQ Create"("Image Name"="untitled") -> ("New Image"=w468:T1, "error out"=w467:errorcluster)  [unwired: 4 in]
          }
          frame "트리거읽기" {
            w479 = T17 2 items=["사용자 홈"=0, "사용자 데스크탑"=1, "사용자 문서"=2, "사용자 어플리케이션 데이터"=3, "사용자 환경"=4, "사용자 임시"=5, "퍼블릭 문서"=6, "퍼블릭 어플리케이션 데이터"=7, "퍼블릭 환경"=8, "퍼블릭 캐시"=13, "시스템 코어 라이브러리"=9, "시스템 설치된 라이브러리"=10, "어플리케이션 파일"=11, "부팅 볼륨 루트"=12] ("system directory type")
            n202 = call <vilib>:"Get System Directory.vi"("system directory type"=w479) -> ("system directory"=w478:path)  [unwired: 10 in]
            n203 = call <vilib>:"IMAQdx Snap2.vi"("error in"=w484, "Image In"=w483, "Session In"=w485) -> ("error out"=w481:errorcluster, "Image Out"=w480:T1, "Session Out"=w482:T15)  [unwired: 6 in]
            n204 = Build Path(base path=w478, name or relative path="test.jpeg") -> ()  [unwired: 1 out]
            n205 = call-poly "IMAQ Write File 2"("File Path"=path "C:/Users/user/Desktop/Labview_final/CNN/Dataset/Color/Test/Test/test.jpeg", "Image"=w480) -> ("error out"=w473:errorcluster, "Image Out (duplicate)"=→"Image 2":T1)  [unwired: 8 in]
            n206 = Unbundle By Name(w476) -> ("CNN"=w475:refnum<queue>)
            n207 = Enqueue Element(queue=w475, element=T4 {"상태"=enum."CNN 통신", "값"=variant} ("원소"), error in (no error)=w473) -> ()  [unwired: 1 in, 3 out]
          }
          frame "닫기" {
            n208 = call <vilib>:"IMAQdx Close Camera.vi"("error in"=w493, "Session In"=w494) -> ("error out"=w490:errorcluster)  [unwired: 9 in]
            n209 = call "IMAQ Dispose"("Image"=w492, "error in (no error)"=w491) -> ("error out"=w488:errorcluster)  [unwired: 4 in]
            n210 = call <vilib>:"Clear Errors.vi"("error in (no error)"=w490) -> ("error out"=w489:errorcluster)  [unwired: 5 in, 1 out]
            n211 = call <vilib>:"Clear Errors.vi"("error in (no error)"=w488) -> ("error out"=w487:errorcluster)  [unwired: 5 in, 1 out]
          }
          frame "프로그램정지" {
            n212 = call <vilib>:"IMAQdx Close Camera.vi"("error in"=w500, "Session In"=w501) -> ("error out"=w503:errorcluster)  [unwired: 9 in]
            n213 = call "IMAQ Dispose"("Image"=w499, "error in (no error)"=w498) -> ("error out"=w502:errorcluster)  [unwired: 4 in]
            n214 = call <vilib>:"Clear Errors.vi"("error in (no error)"=w503) -> ("error out"=w497:errorcluster)  [unwired: 5 in, 1 out]
            n215 = call <vilib>:"Clear Errors.vi"("error in (no error)"=w502) -> ("error out"=w496:errorcluster)  [unwired: 5 in, 1 out]
          }
        }
      }
      frame True {
        n216 = call <vilib>:"IMAQdx Snap2.vi"("error in"=w509, "Image In"=w508, "Session In"=w511) -> ("error out"=w506:errorcluster, "Image Out"=w507:T1, "Session Out"=w510:T15)  [unwired: 6 in]
      }
    }
    "Image" <- w427
    n217 = Wait (ms)(milliseconds to wait=u32 1 ("대기 시간 (ms)")) -> ()  [unwired: 1 out]
  }
